vi "HEWH Set Valves.vi"(0 "VISA session":refnum<visa-resource-name>="MW100", 1 "Valve Bank":u16(ring) items=["A", "B", "C", "D"], 2 "Semiphore":T1, 5 "Expansion Tank?":bool, 7 "Valve Bank Setting":T2, 11 "Error In":errorcluster) -> (4 "dup VISA session":refnum<visa-resource-name>, 15 "Error Out":errorcluster)   [LabVIEW 2012]
uses:
  ValveBankPositions.ctl
  Intellifaucet/Intellfaucet Mode.ctl
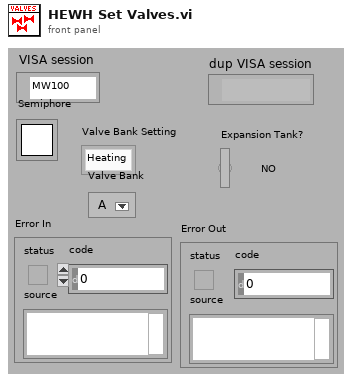
[diagram p1: front panel]
types:
  T1 = typedef "Semaphore RefNum" = refnum<k1>
  T2 = typedef "ValveBankPositions.ctl" = enum16{"Heating", "Purge", "Resting", "Draw"}
  T3 = typedef "Intellfaucet Mode.ctl" = enum16{"Adjust Temp", "Adjust Flow", "Start Flow", "Stop Flow"}
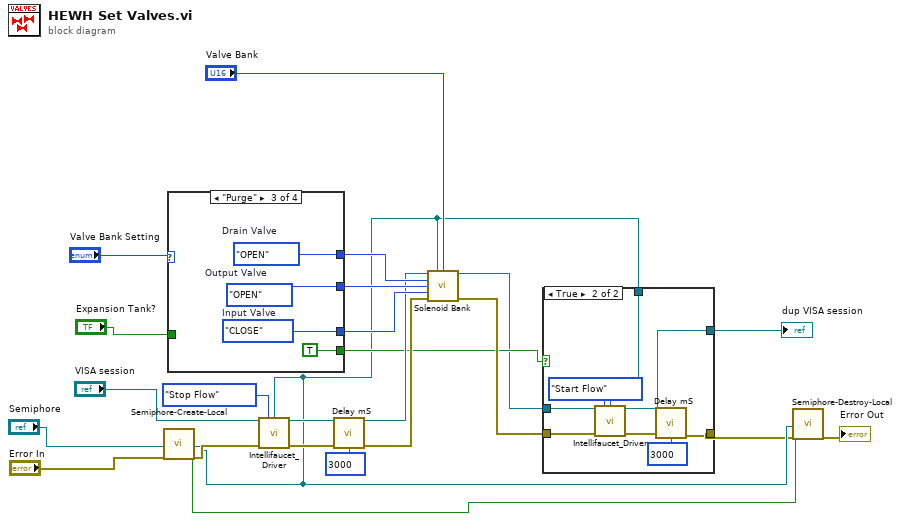
[diagram p0: block diagram]
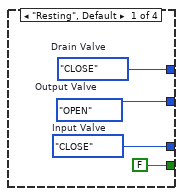
[diagram p3: hidden frame]
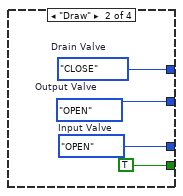
[diagram p4: hidden frame]
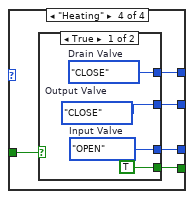
[diagram p5: hidden frame]
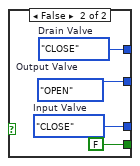
[diagram p6: hidden frame]
diagram:
  n1 = call "Semiphore-Create-Local.vi"("Semiphore"="Semiphore", "error in (no error)"="Error In") -> ("semaphore"=w2:T1, "Local?"=w3:bool, "error out"=w5:errorcluster)  [unwired: 15 in]
  n2 = case shown="\"Purge\"" "Valve Bank Setting" {
    tunnel: [w27 w31 w35 w40] -> w22
    tunnel: [w26 w30 w34 w39] -> w21
    tunnel: [w25 w29 w33 w38] -> w20
    tunnel: "Expansion Tank?" -> [_ _ _ w37]
    tunnel: [FALSE TRUE TRUE w36] -> w10
    frame "Resting", Default {
      w25 = enum8{"OPEN", "CLOSE"}."CLOSE"  # Input Valve
      w26 = enum8{"CLOSE", "OPEN"}."OPEN"  # Output Valve
      w27 = enum8{"OPEN", "CLOSE"}."CLOSE"  # Drain Valve
    }
    frame "Draw" {
      w29 = enum8{"OPEN", "CLOSE"}."OPEN"  # Input Valve
      w30 = enum8{"CLOSE", "OPEN"}."OPEN"  # Output Valve
      w31 = enum8{"OPEN", "CLOSE"}."CLOSE"  # Drain Valve
    }
    frame "Purge" {
      w33 = enum8{"OPEN", "CLOSE"}."CLOSE"  # Input Valve
      w34 = enum8{"CLOSE", "OPEN"}."OPEN"  # Output Valve
      w35 = enum8{"OPEN", "CLOSE"}."OPEN"  # Drain Valve
    }
    frame "Heating" {
      n3 = case shown="True" w37 {
        tunnel: [w44 w48] -> w40
        tunnel: [w43 w47] -> w39
        tunnel: [w42 w46] -> w38
        tunnel: [TRUE FALSE] -> w36
        frame True {
          w42 = enum8{"OPEN", "CLOSE"}."OPEN"  # Input Valve
          w43 = enum8{"CLOSE", "OPEN"}."CLOSE"  # Output Valve
          w44 = enum8{"OPEN", "CLOSE"}."CLOSE"  # Drain Valve
        }
        frame False {
          w46 = enum8{"OPEN", "CLOSE"}."CLOSE"  # Input Valve
          w47 = enum8{"CLOSE", "OPEN"}."OPEN"  # Output Valve
          w48 = enum8{"OPEN", "CLOSE"}."CLOSE"  # Drain Valve
        }
      }
    }
  }
  n4 = call "Intellifaucet_Driver.vi"("VISA session"="VISA session", "Mode"=Intellfaucet_Mode."Stop Flow", "Semiphore"=w2, "Error In"=w5) -> ("VISA session out"=w16:refnum<visa-resource-name>, "Error Out"=w14:errorcluster)  [unwired: 10 in]
  n5 = call "Delay mS.vi"("Error In"=w14, "milliseconds to wait"=u32 3000) -> ("Error Out"=w13:errorcluster)  [unwired: 13 in]
  n6 = call "Solenoid Bank.vi"("VISA session"=w16, "Semiphore"=w2, "Valve Bank"="Valve Bank", "Drain Valve"=w22, "Output Valve"=w21, "Input Valve"=w20, "Error In"=w13) -> ("dup VISA session"=w9:refnum<visa-resource-name>, "Error Out"=w11:errorcluster)  [unwired: 7 in]
  n7 = case shown="True" w10 {
    tunnel: [w50 w51] -> w1
    tunnel: w11 -> [w50 w58]
    tunnel: w9 -> [w49 w56]
    tunnel: [w49 w55] -> w8
    tunnel: w2 -> [_ w54]
    frame False {
    }
    frame True {
      n8 = call "Intellifaucet_Driver.vi"("VISA session"=w56, "Mode"=Intellfaucet_Mode."Start Flow", "Semiphore"=w54, "Error In"=w58) -> ("VISA session out"=w55:refnum<visa-resource-name>, "Error Out"=w52:errorcluster)  [unwired: 10 in]
      n9 = call "Delay mS.vi"("Error In"=w52, "milliseconds to wait"=u32 3000) -> ("Error Out"=w51:errorcluster)  [unwired: 13 in]
    }
  }
  "dup VISA session" <- w8
  n10 = call "Semiphore-Destroy-Local.vi"("Semiphore"=w2, "Local?"=w3, "error in (no error)"=w1) -> ("error out"=→"Error Out":errorcluster)  [unwired: 16 in]
